vi "Execute Spot Correction.vi"(5 "Load Correction (T:Yes)":bool=TRUE, 7 "Short Correction (T:Yes)":bool=TRUE, 8 "error in (no error)":errorcluster, 9 "Open Correction (T:Yes)":bool=TRUE, 10 "Spot No. (1)":i32=1, 11 "VISA resource name":refnum<visa-resource-name>) -> (0 "error out":errorcluster, 3 "VISA resource name out":refnum<visa-resource-name>)   [LabVIEW 2016, in "Agilent E4980.lvlib"]
doc: "Executes open, short and load corrections at the specified measurement point."
uses:
  <instrlib>/Agilent E4980/Agilent E4980.lvlib
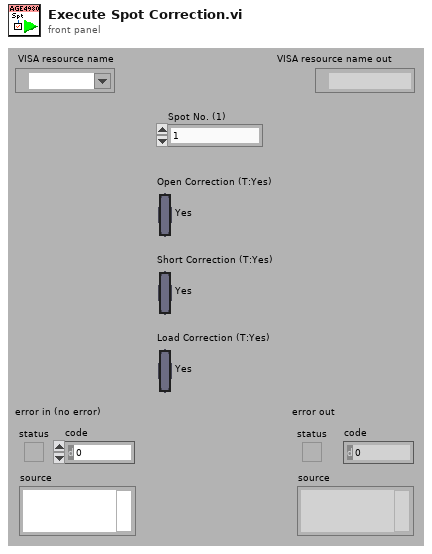
[diagram p1: front panel]
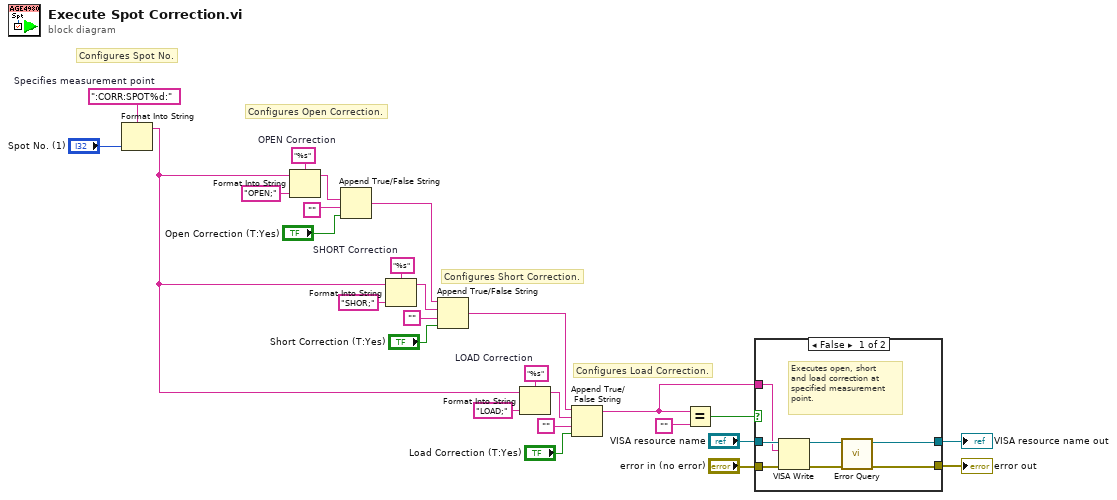
[diagram p0: block diagram]
diagram:
  w15 = "%s"  # LOAD Correction
  w22 = "%s"  # SHORT Correction
  w24 = "%s"  # OPEN Correction
  w27 = ":CORR:SPOT%d:"  # Specifies measurement point
  # "Configures Load Correction."
  # "Configures Short Correction."
  # "Configures Open Correction."
  # "Configures Spot No."
  n1 = Format Into String(format string=w27, "Spot No. (1)") -> (resulting string=w10:string)  [unwired: 2 in, 1 out]
  n2 = Format Into String(format string=w24, initial string=w10, "OPEN;" ("input 1")) -> (resulting string=w1:string)  [unwired: 1 in, 1 out]
  n3 = Append True/False String(1:"Open Correction (T:Yes)", 2:"" ("Empty String Constant"), 3:w1) -> (0:w4:string)  [unwired: 1 in]
  n4 = Format Into String(format string=w22, initial string=w10, "SHOR;" ("input 1")) -> (resulting string=w20:string)  [unwired: 1 in, 1 out]
  n5 = Append True/False String(1:"Short Correction (T:Yes)", 2:"" ("Empty String Constant"), 3:w20, 4:w4) -> (0:w3:string)
  n6 = Format Into String(format string=w15, initial string=w10, "LOAD;" ("input 1")) -> (resulting string=w17:string)  [unwired: 1 in, 1 out]
  n7 = Append True/False String(1:"Load Correction (T:Yes)", 2:"" ("Empty String Constant"), 3:w17, 4:w3) -> (0:w2:string)
  n8 = Equal?(x=w2, y="" ("Empty String Constant")) -> (x = y?=w6:bool)
  n9 = case shown="False" w6 {
    tunnel: "VISA resource name" -> [w32 w36]
    tunnel: "error in (no error)" -> [w31 w35]
    tunnel: [w30 w36] -> w9
    tunnel: [w29 w35] -> w8
    tunnel: w2 -> [w28 _]
    frame False {
      # "Executes open, short\nand load correction at\nspecified measurement\npoint."
      n10 = VISA Write(VISA resource name=w32, write buffer=w28, error in (no error)=w31) -> (VISA resource name out=w33:refnum<visa-resource-name>, error out=w34:errorcluster)  [unwired: 1 out]
      n11 = call <instrlib>:"Error Query.vi"("error in (no error)"=w34, "VISA resource name"=w33) -> ("error out"=w29:errorcluster, "VISA resource name out"=w30:refnum<visa-resource-name>)  [unwired: 6 in, 2 out]
    }
    frame True {
      # "Doesn't send anything\nto the instrument."
    }
  }
  "error out" <- w8
  "VISA resource name out" <- w9
